vi "[Version] - Get Application Main.vi"() -> (0 "Version":string)   [LabVIEW 2016]
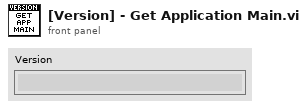
[diagram p1: front panel]
types:
  T1 = enum32{"invalid app kind", "Development System", "Run Time System", "Student Edition", "Embedded LabVIEW", "Evaluation", "Custom"}
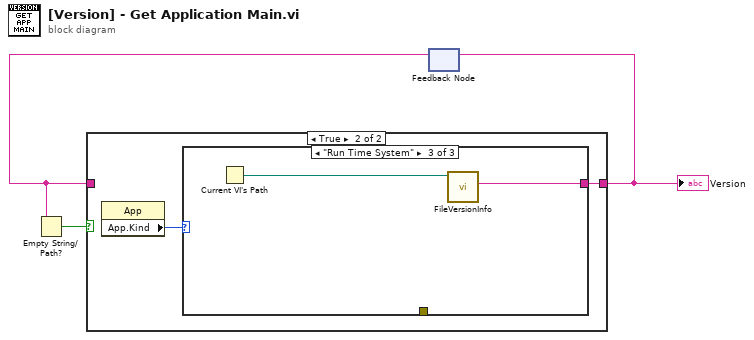
[diagram p0: block diagram]
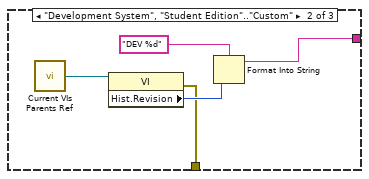
[diagram p4: hidden frame]
diagram:
  n1 = feedback #1() -> (w2:string)  [unwired: 1 in]
  n2 = Empty String/Path?(string/path=w2) -> (empty?=w1:bool)
  n3 = case shown="True" w1 {
    tunnel: [w4 w5] -> w3
    tunnel: w2 -> [w4 _]
    frame False {
    }
    frame True {
      n4 = property class="App"() -> ("App.Kind"=w6:T1)  [unwired: 2 in, 2 out]
      n5 = case shown="\"Run Time System\"" w6 {
        tunnel: [_ w9 w13] -> w5
        tunnel: [_ w7 _] -> _
        frame "invalid app kind" {
        }
        frame "Development System", "Student Edition".."Custom" {
          n6 = call "Current VIs Parents Ref.vi"() -> ("Calling VI's reference"=w8:refnum<vi>)  [unwired: 2 in]
          n7 = property class="VI"(reference=w8) -> (error out=w7:errorcluster, "Hist.Revision"=w11:u32)  [unwired: 1 in, 1 out]
          n8 = Format Into String(format string="DEV %d", w11) -> (resulting string=w9:string)  [unwired: 2 in, 1 out]
        }
        frame "Run Time System" {
          n9 = Current VI's Path() -> (path=w12:path)
          n10 = call <vilib>:"FileVersionInfo.vi"("Application Path in"=w12) -> ("File Version Info"=w13:string)  [unwired: 7 in, 3 out]
        }
      }
    }
  }
  "Version" <- w3
  n11 = feedback-in #1(w3) -> ()
